vi "SRV_Add_C_Line.vi"(3 "inc":i32, 4 "C String":string, 5 "SuperPro in":T1) -> (2 "SuperPro out":T1)   [LabVIEW 2009]
uses:
  <userlib>/SuperPro/OpCodes/_SubVIs/SuperProControl.ctl
panel:
  # "This LabVIEW item is deprecated.\n\nIt is believed to be unused and will be removed in a future version of SRV."
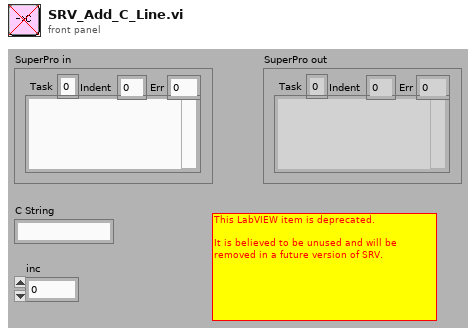
[diagram p1: front panel]
types:
  T1 = typedef "SuperProControl.ctl" = cluster{"Task":i32, "Indent":i32, "Err":i32, "ASM":string}
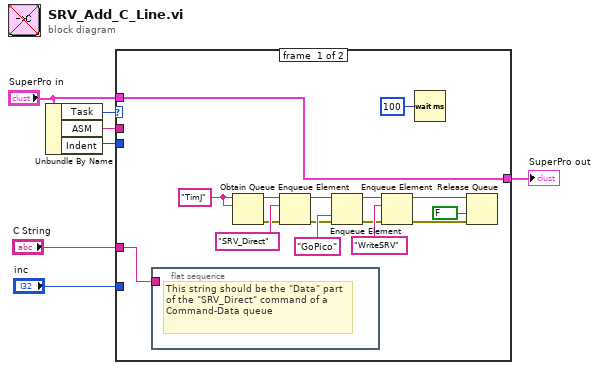
[diagram p0: block diagram]
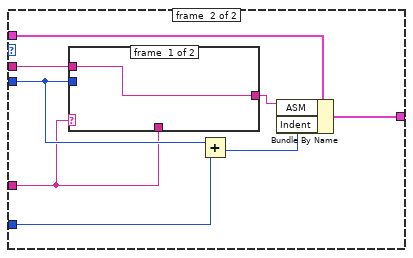
[diagram p2: hidden frame]
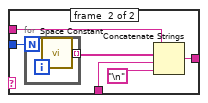
[diagram p3: hidden frame]
diagram:
  n1 = Unbundle By Name("SuperPro in") -> ("Task"=w1:i32, "ASM"=w7:string, "Indent"=w5:i32)
  n2 = case shown="-1" w1 {
    tunnel: w7 -> [_ w31]
    tunnel: "inc" -> [_ w29]
    tunnel: w5 -> [_ w28]
    tunnel: [w23 w27] -> w4
    tunnel: "SuperPro in" -> [w23 w26]
    tunnel: "C String" -> [w14 w24]
    frame #0 {
      w21 = "TimJ" ("name (unnamed)")
      n3 = flat-sequence {
        tunnel: w14 -> [_]
        frame #0 {
          # "This string should be the \"Data\" part of the \"SRV_Direct\" command of a Command-Data queue"
        }
      }
      n4 = Obtain Queue(name (unnamed)=w21, element data type=w21) -> (queue out=w22:refnum<queue>, error out=w12:errorcluster)  [unwired: 3 in, 1 out]
      n5 = Enqueue Element(queue=w22, element="SRV_Direct" ("name (unnamed)"), error in (no error)=w12) -> (queue out=w17:refnum<queue>, error out=w11:errorcluster)  [unwired: 1 in, 1 out]
      n6 = Enqueue Element(queue=w17, element="GoPico" ("name (unnamed)"), error in (no error)=w11) -> (queue out=w19:refnum<queue>, error out=w10:errorcluster)  [unwired: 1 in, 1 out]
      n7 = Enqueue Element(queue=w19, element="WriteSRV" ("name (unnamed)"), error in (no error)=w10) -> (queue out=w13:refnum<queue>, error out=w9:errorcluster)  [unwired: 1 in, 1 out]
      n8 = Wait (ms)(milliseconds to wait=u32 100) -> ()  [unwired: 1 out]
      n9 = Release Queue(queue=w13, force destroy? (F)=FALSE, error in (no error)=w9) -> ()  [unwired: 3 out]
    }
    frame #1 {
      n10 = case shown="Default" w24 {
        tunnel: w31 -> [w32 w38]
        tunnel: [w32 w37] -> w30
        tunnel: w24 -> [_ w36]
        tunnel: w28 -> [_ w33]
        frame #0 {
        }
        frame #1 {
          n11 = for {
            N: w33 -> [_]
            tunnel: [w39] -> w34 mode=indexing
            n12 = call <vilib>:"Space Constant.vi"() -> ("String"=w39:string)
          }
          n13 = Concatenate Strings(w38, w34, w36, "\n") -> (w37:string)
        }
      }
      n14 = Add(x=w28, y=w29) -> (x+y=w25:i32)
      n15 = Bundle By Name(cluster=w26, "ASM"=w30, "Indent"=w25) -> (w27:T1)
    }
  }
  "SuperPro out" <- w4
